vi "Run All.vi"(8 "Error In":errorcluster) -> (0 "Error Out":errorcluster)   [LabVIEW 2018, in "Tests.lvlib" / "Nodes.lvlib"]
uses:
  Nodes.lvlib
  <vilib>/addons/_JKI Toolkits/Caraya/classes/Test/Test.lvclass
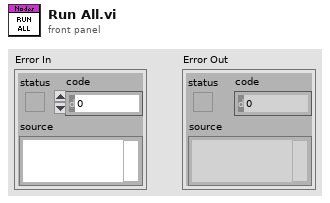
[diagram p1: front panel]
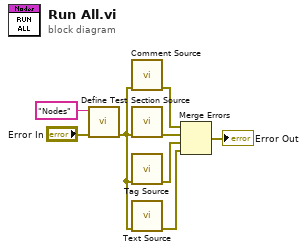
[diagram p0: block diagram]
diagram:
  n1 = call <vilib>:"Define Test.vi"("error in (no error)"="Error In", "Label (VI Title)"="Nodes") -> ("error out"=w2:errorcluster)  [unwired: 9 in]
  n2 = call "Comment Source.vi"("Error In"=w2) -> ("Error Out"=w6:errorcluster)  [unwired: 10 in]
  n3 = call "Section Source.vi"("Error In"=w2) -> ("Error Out"=w5:errorcluster)  [unwired: 10 in]
  n4 = call "Tag Source.vi"("Error In"=w2) -> ("Error Out"=w3:errorcluster)  [unwired: 10 in]
  n5 = call "Text Source.vi"("Error In"=w2) -> ("Error Out"=w1:errorcluster)  [unwired: 10 in]
  n6 = Merge Errors(w6, w5, w3, w1) -> (→"Error Out":errorcluster)
